vi "DS345 Write.vi"(2 "ON or OFF?":bool[](array[boolean])=[TRUE, TRUE, FALSE], 3 "error in":errorcluster, 4 "Interval Lengths (ms)":dbl[](array[numeric])=[70.0, 30.0, 10.0] format="%.3f", 5 "Arbitrary Waveform Array of Channels (only uses CH 0)":T1(array[cluster])=[[{"AC Frequency (kHz)"=10.0, " Initial AC Ampl. (p-p/2)"=5.0, "Final AC Ampl."=0.0, "Initial DC Value"=-0.1, "Final DC Value"=-0.04, "Constant"=240.0, "Gamma AC"=1.0, "String"="Channel 0 A", "Gamma DC"=0.0}, {"AC Frequency (kHz)"=10.0, " Initial AC Ampl. (p-p/2)"=0.0, "Final AC Ampl."=0.0, "Initial DC Value"=-0.1, "Final DC Value"=-0.04, "Constant"=240.0, "Gamma AC"=1.0, "String"="Channel 0 B", "Gamma DC"=0.0}, {"AC Frequency (kHz)"=10.0, " Initial AC Ampl. (p-p/2)"=0.0, "Final AC Ampl."=0.0, "Initial DC Value"=-0.1, "Final DC Value"=-0.04, "Constant"=240.0, "Gamma AC"=1.0, "String"="Channel 0 C", "Gamma DC"=0.0}], [{"AC Frequency (kHz)"=10.0, " Initial AC Ampl. (p-p/2)"=5.0, "Final AC Ampl."=0.0, "Initial DC Value"=-0.1, "Final DC Value"=-0.04, "Constant"=240.0, "Gamma AC"=1.0, "String"="Channel 1 A", "Gamma DC"=0.0}, {"AC Frequency (kHz)"=10.0, " Initial AC Ampl. (p-p/2)"=0.0, "Final AC Ampl."=0.0, "Initial DC Value"=-0.1, "Final DC Value"=-0.04, "Constant"=199.2, "Gamma AC"=1.0, "String"="Channel 1 B", "Gamma DC"=0.0}, {"AC Frequency (kHz)"=10.0, " Initial AC Ampl. (p-p/2)"=0.0, "Final AC Ampl."=0.0, "Initial DC Value"=-0.1, "Final DC Value"=-0.04, "Constant"=199.2, "Gamma AC"=1.0, "String"="Channel 1 C", "Gamma DC"=0.0}], [{"AC Frequency (kHz)"=10.0, " Initial AC Ampl. (p-p/2)"=0.0, "Final AC Ampl."=0.0, "Initial DC Value"=-0.1, "Final DC Value"=-0.04, "Constant"=199.2, "Gamma AC"=1.0, "String"="Channel 2 A", "Gamma DC"=0.0}, {"AC Frequency (kHz)"=10.0, " Initial AC Ampl. (p-p/2)"=0.0, "Final AC Ampl."=0.0, "Initial DC Value"=-0.1, "Final DC Value"=-0.04, "Constant"=199.2, "Gamma AC"=1.0, "String"="Channel 2 B", "Gamma DC"=0.0}, {"AC Frequency (kHz)"=10.0, " Initial AC Ampl. (p-p/2)"=0.0, "Final AC Ampl."=0.0, "Initial DC Value"=-0.1, "Final DC Value"=-0.04, "Constant"=199.2, "Gamma AC"=1.0, "String"="Channel 2 C", "Gamma DC"=0.0}], [{"AC Frequency (kHz)"=10.0, " Initial AC Ampl. (p-p/2)"=0.0, "Final AC Ampl."=0.0, "Initial DC Value"=-0.1, "Final DC Value"=-0.04, "Constant"=199.2, "Gamma AC"=1.0, "String"="Channel 3 A", "Gamma DC"=0.0}, {"AC Frequency (kHz)"=10.0, " Initial AC Ampl. (p-p/2)"=0.0, "Final AC Ampl."=0.0, "Initial DC Value"=-0.1, "Final DC Value"=-0.04, "Constant"=199.2, "Gamma AC"=1.0, "String"="Channel 3 B", "Gamma DC"=0.0}, {"AC Frequency (kHz)"=10.0, " Initial AC Ampl. (p-p/2)"=0.0, "Final AC Ampl."=0.0, "Initial DC Value"=-0.1, "Final DC Value"=-0.04, "Constant"=199.2, "Gamma AC"=1.0, "String"="Channel 3 C", "Gamma DC"=0.0}], [{"AC Frequency (kHz)"=10.0, " Initial AC Ampl. (p-p/2)"=0.0, "Final AC Ampl."=0.0, "Initial DC Value"=-0.1, "Final DC Value"=-0.04, "Constant"=199.2, "Gamma AC"=1.0, "String"="Channel 4 A", "Gamma DC"=0.0}, {"AC Frequency (kHz)"=10.0, " Initial AC Ampl. (p-p/2)"=0.0, "Final AC Ampl."=0.0, "Initial DC Value"=-0.1, "Final DC Value"=-0.04, "Constant"=199.2, "Gamma AC"=1.0, "String"="Channel 4 B", "Gamma DC"=0.0}, {"AC Frequency (kHz)"=10.0, " Initial AC Ampl. (p-p/2)"=0.0, "Final AC Ampl."=0.0, "Initial DC Value"=-0.1, "Final DC Value"=-0.04, "Constant"=199.2, "Gamma AC"=1.0, "String"="Channel 4 C", "Gamma DC"=0.0}], [{"AC Frequency (kHz)"=10.0, " Initial AC Ampl. (p-p/2)"=0.0, "Final AC Ampl."=0.0, "Initial DC Value"=-0.1, "Final DC Value"=-0.04, "Constant"=199.2, "Gamma AC"=1.0, "String"="Channel 5 A", "Gamma DC"=0.0}, {"AC Frequency (kHz)"=10.0, " Initial AC Ampl. (p-p/2)"=0.0, "Final AC Ampl."=0.0, "Initial DC Value"=-0.1, "Final DC Value"=-0.04, "Constant"=199.2, "Gamma AC"=1.0, "String"="Channel 5 B", "Gamma DC"=0.0}, {"AC Frequency (kHz)"=10.0, " Initial AC Ampl. (p-p/2)"=0.0, "Final AC Ampl."=0.0, "Initial DC Value"=-0.1, "Final DC Value"=-0.04, "Constant"=199.2, "Gamma AC"=1.0, "String"="Channel 5 C", "Gamma DC"=0.0}], [{"AC Frequency (kHz)"=10.0, " Initial AC Ampl. (p-p/2)"=0.0, "Final AC Ampl."=0.0, "Initial DC Value"=-0.1, "Final DC Value"=-0.04, "Constant"=199.2, "Gamma AC"=1.0, "String"="Channel 6 A", "Gamma DC"=0.0}, {"AC Frequency (kHz)"=10.0, " Initial AC Ampl. (p-p/2)"=0.0, "Final AC Ampl."=0.0, "Initial DC Value"=-0.1, "Final DC Value"=-0.04, "Constant"=199.2, "Gamma AC"=1.0, "String"="Channel 6 B", "Gamma DC"=0.0}, {"AC Frequency (kHz)"=10.0, " Initial AC Ampl. (p-p/2)"=0.0, "Final AC Ampl."=0.0, "Initial DC Value"=-0.1, "Final DC Value"=-0.04, "Constant"=199.2, "Gamma AC"=1.0, "String"="Channel 6 C", "Gamma DC"=0.0}], [{"AC Frequency (kHz)"=10.0, " Initial AC Ampl. (p-p/2)"=0.0, "Final AC Ampl."=0.0, "Initial DC Value"=-0.1, "Final DC Value"=-0.04, "Constant"=199.2, "Gamma AC"=1.0, "String"="Channel 7 A", "Gamma DC"=0.0}, {"AC Frequency (kHz)"=10.0, " Initial AC Ampl. (p-p/2)"=0.0, "Final AC Ampl."=0.0, "Initial DC Value"=-0.1, "Final DC Value"=-0.04, "Constant"=199.2, "Gamma AC"=1.0, "String"="Channel 7 B", "Gamma DC"=0.0}, {"AC Frequency (kHz)"=10.0, " Initial AC Ampl. (p-p/2)"=0.0, "Final AC Ampl."=0.0, "Initial DC Value"=-0.1, "Final DC Value"=-0.04, "Constant"=199.2, "Gamma AC"=1.0, "String"="Channel 7 C", "Gamma DC"=0.0}]] {"Gamma DC" format="%.2f"; "Gamma AC" format="%.2f"; "Constant" min=0.0 max=240.0 format="%.2f"; "Final DC Value" format="%.3f"; "Initial DC Value" format="%.3f"; "Final AC Ampl." format="%.3f"; "Initial AC Ampl. (p-p/2)" format="%.3f"; "AC Frequency (kHz)" format="%.2f"}) -> (0 "error out":errorcluster, 1 "Waveform (dither)":cluster{dbl[], dbl[]}(graph))   [LabVIEW 2013]
panel:
  in  "Case Constant\n(See Context Help)":bool=TRUE
  out "Actual used channels":bool[](array[boolean])
  out "Array":dbl[](array[numeric]) format="%^.5e"
  out "log2(x)":dbl format="%.2f"
  out "ceil(x): smallest int >= x":dbl format="%.2f"
  out "Est. Sampling Rate":dbl format="%.2f"
  out "Total Waveform Time":dbl format="%.2f"
  out "Number of points":dbl=16000.0 format="%.2f"
  out "Sampling Rate":dbl=160000.0 format="%.2f"
  in  "trigger rate":ext=100.0 format="%.3f"
  in  "Memory Address (0 to 9)\n(stores waveform)":string="0"
  in  "trigger source (single:0)":i32(ring)=2 items=["single", "internal rate", "+ slope external", "- slope external", "line"]
  in  "ARB.wave source":u16(ring)=1 items=[".WAV file", "array in point mode", "array in vector mode"]
  in  "single trigger":bool
  in  "FREQ. units (Hz:0)":i32(ring) items=["Hz", "KHz.", "MHz."]
  in  "phase":ext format="%.3f"
  in  "DC offset":ext format="%.3f"
  in  "amplitude (0 Vrms:0)":cluster{ext, i32}={1.0, 1} {"?" items=["Vrms", "Vpp", "dBm"]; "?" format="%.3f"}
  in  "frequency":ext=555.0 format="%.6f"
  in  "output function (sine:0)":u16(ring)=5 items=["sine", "square", "triangle", "ramp", "noise", "arbitrary"]
  in  "Command to Send":string="*RST;"
  in  "GPIB Address":string="19"
  # "DS 345 Settings"
  # "Note that Interval C is disabled for DS345"
  # "Sampling Rate of DS345\nDefaults to Closest Value \n(up or down) of \n40MHz/n where n is a\npositive integer."
  # "Interval A"
  # "Interval B"
  # "Interval C"
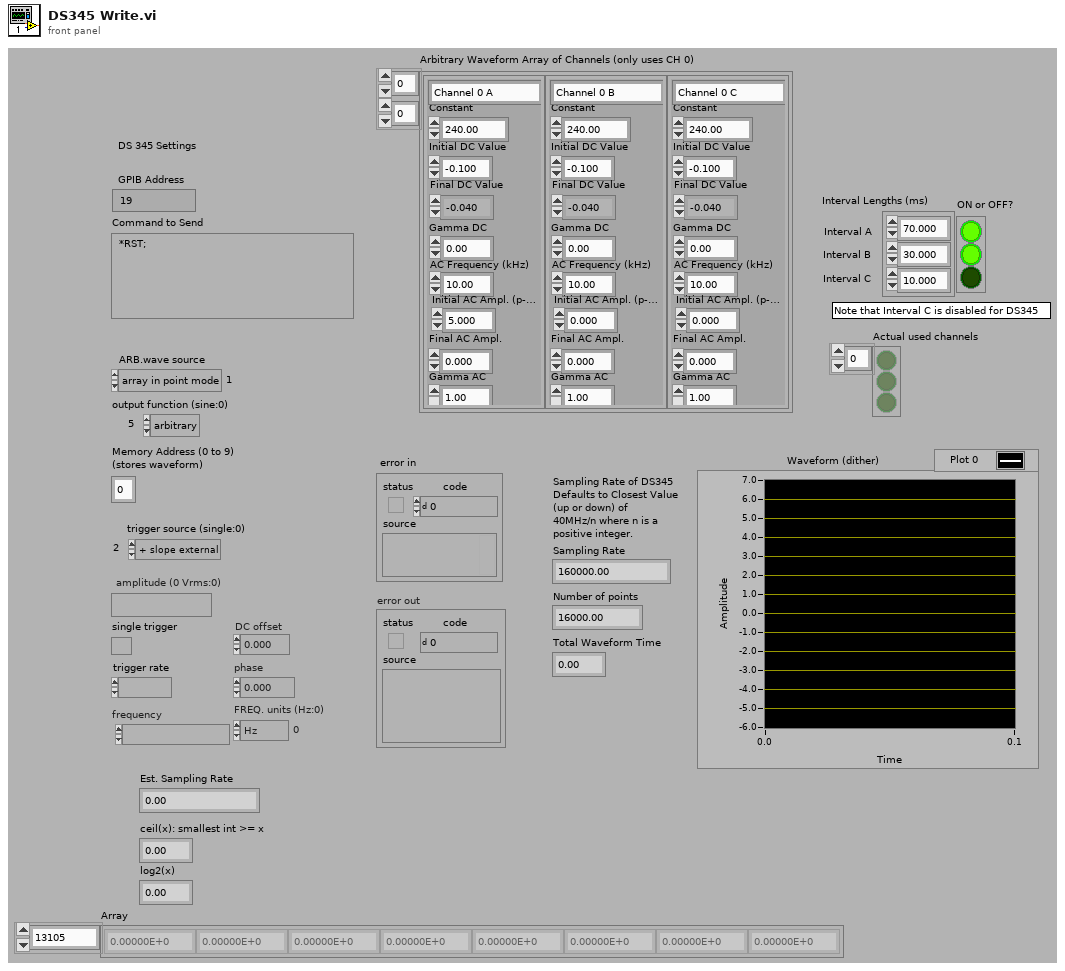
[diagram p1: front panel]
types:
  T1 = cluster{"AC Frequency (kHz)":dbl, " Initial AC Ampl. (p-p/2)":dbl, "Final AC Ampl.":dbl, "Initial DC Value":dbl, "Final DC Value":dbl, "Constant":dbl, "Gamma AC":dbl, "String":string, "Gamma DC":dbl}[][]
  T2 = cluster{"AC Frequency (kHz)":dbl, " Initial AC Ampl. (p-p/2)":dbl, "Final AC Ampl.":dbl, "Initial DC Value":dbl, "Final DC Value":dbl, "Constant":dbl, "Gamma AC":dbl, "String":string, "Gamma DC":dbl}[]
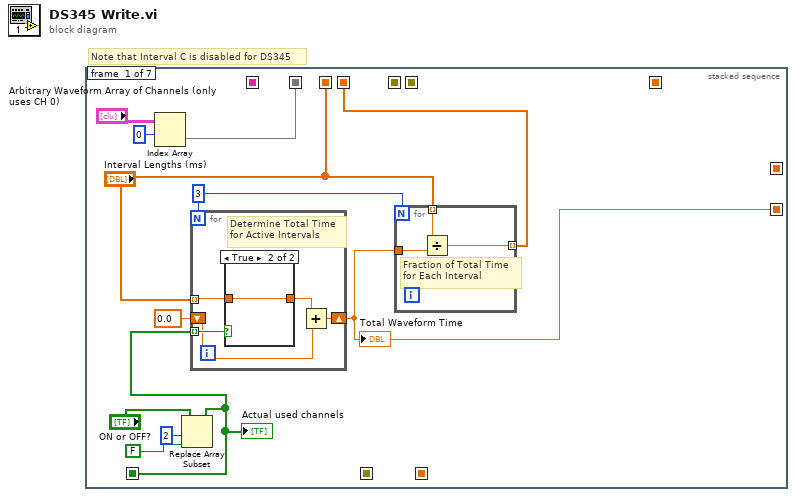
[diagram p0: block diagram]
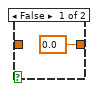
[diagram p2: hidden frame]
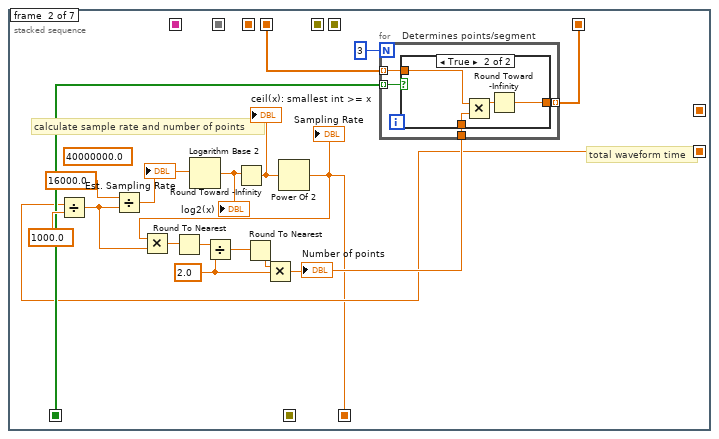
[diagram p3: hidden frame]
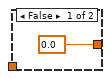
[diagram p4: hidden frame]
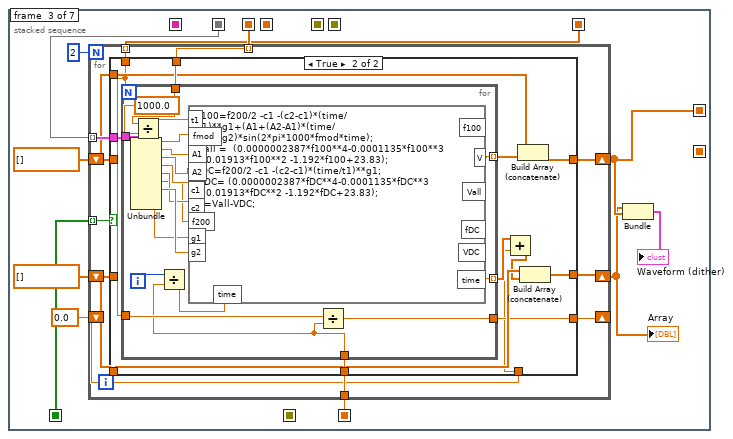
[diagram p5: hidden frame]
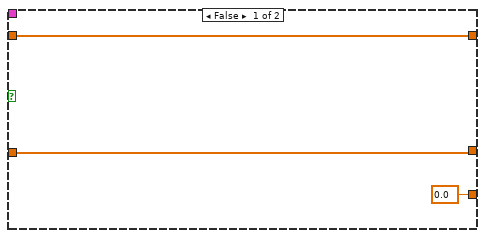
[diagram p6: hidden frame]
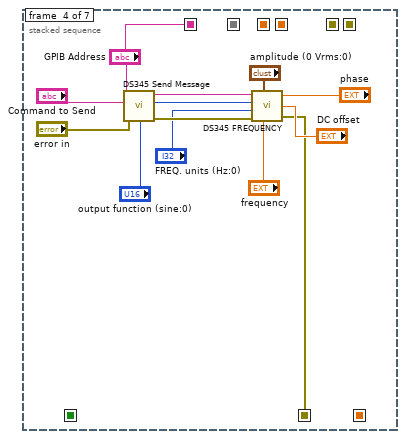
[diagram p7: hidden frame]
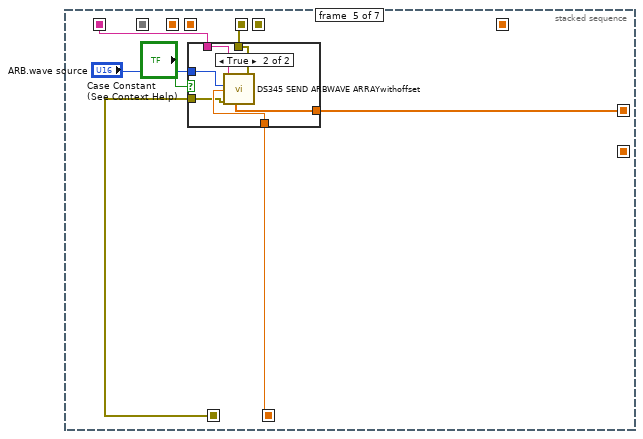
[diagram p8: hidden frame]
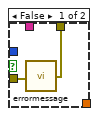
[diagram p9: hidden frame]
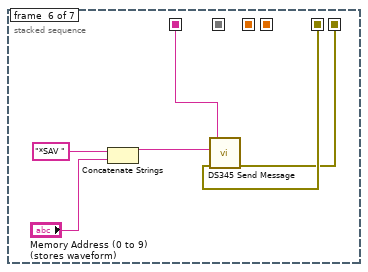
[diagram p10: hidden frame]
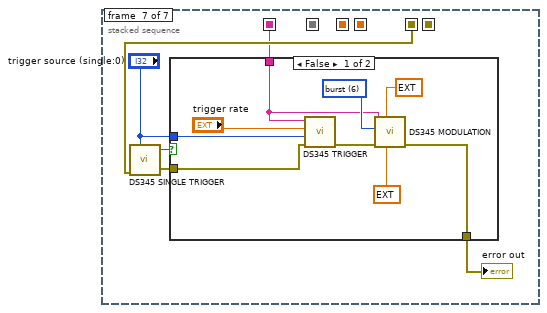
[diagram p11: hidden frame]
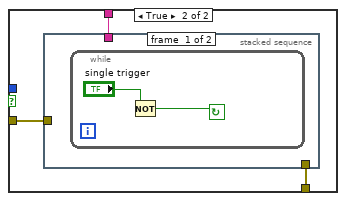
[diagram p12: hidden frame]
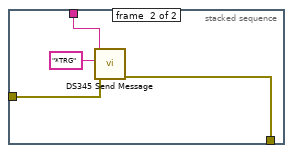
[diagram p13: hidden frame]
diagram:
  # "Note that Interval C is disabled for DS345"
  n1 = stacked-sequence {
    seq-local: [_ _ _ _ w125 _ _] -> [_ _ _ _ _ w137 w145]
    seq-local: [_ _ _ _ _ w136 _] -> [_ _ _ _ _ _ _]
    seq-local: [_ w23 _ _ _ _ _] -> [_ _ w61 _ w120 _ _]
    seq-local: [_ _ w52 _ _ _ _] -> [_ _ _ _ w121 _ _]
    seq-local: [_ _ _ "GPIB Address" _ _ _] -> [_ _ _ _ w123 w135 w142]
    seq-local: [_ _ _ w108 _ _ _] -> [_ _ _ _ w122 _ _]
    seq-local: [w11 _ _ _ _ _ _] -> [_ _ w60 _ _ _ _]
    seq-local: [w5 _ _ _ _ _ _] -> [_ w28 _ _ _ _ _]
    seq-local: ["Interval Lengths (ms)" _ _ _ _ _ _] -> [_ _ w59 _ _ _ _]
    seq-local: [w6 _ _ _ _ _ _] -> [_ w30 _ _ _ _ _]
    seq-local: [_ w31 _ _ _ _ _] -> [_ _ w58 _ _ _ _]
    seq-local: [w1 _ _ _ _ _ _] -> [_ w32 w56 _ _ _ _]
    frame #0 {
      w9 = 3
      n2 = Index Array(array="Arbitrary Waveform Array of Channels (only uses CH 0)", index (row)=0) -> (element=w11:T2)  [unwired: 1 in]
      n3 = Replace Array Subset(array="ON or OFF?", new element=FALSE ("new element/subarray"), index=2) -> (w1:bool[])
      "Actual used channels" <- w1
      n4 = for {
        N: w9 -> [_]
        tunnel: w1 -> [w20] mode=indexing
        tunnel: "Interval Lengths (ms)" -> [w19] mode=indexing
        shift-right: [w17] -> w5
        shift-left: 0.0 -> [w16]
        # "Determine Total Time\nfor Active Intervals"
        n5 = case shown="True" w20 {
          tunnel: w19 -> [_ w22]
          tunnel: [0.0 ("Interval A (ms)") w22] -> w18
          frame False {
          }
          frame True {
          }
        }
        n6 = Add(x=w18, y=w16) -> (x+y=w17:dbl)
      }
      "Total Waveform Time" <- w5
      n7 = for {
        N: w9 -> [_]
        tunnel: "Interval Lengths (ms)" -> [w15] mode=indexing
        tunnel: w5 -> [w14]
        tunnel: [w13] -> w6 mode=indexing
        # "Fraction of Total Time\nfor Each Interval"
        n8 = Divide(x=w15, y=w14) -> (x/y=w13:dbl)
      }
    }
    frame #1 {
      w34 = 2.0 ("y")
      (unwired) 40000000.0 ("x")
      # "total waveform time"
      # "calculate sample rate and number of points"
      n9 = Divide(x=w28, y=1000.0 ("10000")) -> (x/y=w27:dbl)
      n10 = Divide(x=16000.0, y=w27) -> (x/y=w26:dbl)
      "Est. Sampling Rate" <- w26
      n11 = Logarithm Base 2(1:w26) -> (0:w25:dbl)
      "log2(x)" <- w25
      n12 = Round Toward -Infinity(1:w25) -> (0:w24:dbl)
      "ceil(x): smallest int >= x" <- w24
      n13 = Power Of 2(x=w24) -> (2^x=w23:dbl)
      "Sampling Rate" <- w23
      n14 = Multiply(x=w23, y=w27) -> (x*y=w38:dbl)
      n15 = Round To Nearest(number=w38) -> (nearest integer value=w37:dbl)
      n16 = Divide(x=w37, y=w34) -> (x/y=w36:dbl)
      n17 = Round To Nearest(number=w36) -> (nearest integer value=w35:dbl)
      n18 = Multiply(x=w35, y=w34) -> (x*y=w33:dbl)
      "Number of points" <- w33
      n19 = for "Determines points/segment" {
        N: 3 -> [_]
        tunnel: w32 -> [w44] mode=indexing
        tunnel: [w43] -> w31 mode=indexing
        tunnel: w33 -> [w42]
        tunnel: w30 -> [w41] mode=indexing
        n20 = case shown="True" w44 {
          tunnel: [0.0 w49] -> w43
          tunnel: w42 -> [_ w47]
          tunnel: w41 -> [_ w46]
          frame False {
          }
          frame True {
            n21 = Multiply(x=w46, y=w47) -> (x*y=w48:dbl)
            n22 = Round Toward -Infinity(1:w48) -> (0:w49:dbl)
          }
        }
      }
    }
    frame #2 {
      n23 = for {
        N: 2 -> [_]
        tunnel: w61 -> [w72]
        tunnel: w60 -> [w71] mode=indexing
        tunnel: w59 -> [w70] mode=indexing
        tunnel: w58 -> [w69] mode=indexing
        tunnel: w56 -> [w68] mode=indexing
        shift-right: [w67] -> w52
        shift-left: dbl[] [] -> [w66]
        shift-right: [w65] -> w51
        shift-left: dbl[] [] -> [w64]
        shift-right: [w63] -> _
        shift-left: 0.0 -> [w62]
        n24 = case shown="True" w68 {
          tunnel: w72 -> [_ w88]
          tunnel: w71 -> [_ w87]
          tunnel: w70 -> [_ w86]
          tunnel: w69 -> [_ w80]
          tunnel: [w75 w84] -> w67
          tunnel: w66 -> [_ w83]
          tunnel: w66 -> [w75 _]
          tunnel: [w74 w82] -> w65
          tunnel: w64 -> [_ w81]
          tunnel: w64 -> [w74 _]
          tunnel: [0.0 w79] -> w63
          tunnel: w62 -> [_ w77]
          frame False {
          }
          frame True {
            n25 = for {
              N: w80 -> [_]
              tunnel: w88 -> [w90]
              tunnel: w87 -> [w106]
              tunnel: w86 -> [w102]
              tunnel: [w97] -> w85 mode=indexing
              tunnel: [w96] -> w78 mode=indexing
              tunnel: w80 -> [w91]
              tunnel: [w89] -> w79
              i -> [w107]
              n26 = Unbundle(w106) -> ("AC Frequency (kHz)"=w98:dbl, "Initial AC Ampl. (p-p/2)"=w99:dbl, "Final AC Ampl."=w100:dbl, "Initial DC Value"=w95:dbl, "Final DC Value"=w94:dbl, "Constant"=w93:dbl, "Gamma AC"=w101:dbl, "Gamma DC"=w92:dbl)  [unwired: 1 out]
              n27 = Divide(x=w102, y=1000.0) -> (x/y=w103:dbl)
              n28 = Divide(x=w107, y=w90) -> (x/y=w105:dbl)
              n29 = formula code="f100=f200/2 -c1 -(c2-c1)*(time/t1)**g1+(A1+(A2-A1)*(time/t1)**g2)*sin(2*pi*1000*fmod*time);\nVall =  (0.0000002387*f100**4-0.0001135*f100**3 +0.01913*f100**2 -1.192*f100+23.83);\nfDC=f200/2 -c1 -(c2-c1)*(time/t1)**g1;\nVDC= (0.0000002387*fDC**4-0.0001135*fDC**3 +0.01913*fDC**2 -1.192*fDC+23.83);\nV=Vall-VDC;"("c1"=w95, "time"=w105, "t1"=w103, "c2"=w94, "f200"=w93, "fmod"=w98, "A1"=w99, "A2"=w100, "g1"=w92, "g2"=w101) -> ("time"=w96:dbl, "V"=w97:dbl)  [unwired: 4 out]
              n30 = Divide(x=w91, y=w90) -> (x/y=w89:dbl)
            }
            n31 = Add(x=w78, y=w77) -> (x+y=w76:dbl[])
            n32 = Build Array (concatenate)(w83, w85) -> (w84:dbl[])
            n33 = Build Array (concatenate)(w81, w76) -> (w82:dbl[])
          }
        }
      }
      "Array" <- w51
      n34 = Bundle(w51, w52) -> (→"Waveform (dither)":cluster{dbl[], dbl[]})  [unwired: 1 in]
    }
    frame #3 {
      n35 = call "DS345 Send Message.vi"("address string"="GPIB Address", "write buffer"="Command to Send", "error in"="error in") -> ("address out"=w110:string, "error out"=w114:errorcluster)  [unwired: 3 in, 2 out]
      n36 = call "DS345 FREQUENCY.vi"("GPIB address"=w110, "amplitude (0 Vrms:0)"="amplitude (0 Vrms:0)", "output function (sine:0)"="output function (sine:0)", "FREQ. units (Hz:0)"="FREQ. units (Hz:0)", "frequency"="frequency", "error in"=w114, "phase"="phase", "DC offset"="DC offset") -> ("error out"=w108:errorcluster)
    }
    frame #4 {
      n37 = case shown="True" "Case Constant\n(See Context Help)" {
        tunnel: "ARB.wave source" -> [_ w134]
        tunnel: w123 -> [_ w133]
        tunnel: [w128 w132] -> w125
        tunnel: w120 -> [_ w131]
        tunnel: w122 -> [w127 w130]
        tunnel: w121 -> [_ w129]
        frame False {
          n38 = call "errormessage.vi"("error in"=w127) -> ("error out"=w128:errorcluster)
        }
        frame True {
          n39 = call "DS345 SEND ARBWAVE ARRAYwithoffset.VI"("y vertices / amplitude points"=w129, "error in"=w130, "sampling FREQ."=w131, "ARB.wave source"=w134, "GPIB address"=w133) -> ("error out"=w132:errorcluster)  [unwired: 1 in]
        }
      }
    }
    frame #5 {
      n40 = Concatenate Strings("*SAV " ("string"), "Memory Address (0 to 9)\n(stores waveform)") -> (w138:string)
      n41 = call "DS345 Send Message.vi"("address string"=w135, "write buffer"=w138, "error in"=w137) -> ("error out"=w136:errorcluster)  [unwired: 3 in, 3 out]
    }
    frame #6 {
      n42 = call "DS345 SINGLE TRIGGER.VI"("error in"=w145, "trigger source (single:0)"="trigger source (single:0)") -> ("error out"=w141:errorcluster, "single trigger"=w146:bool)  [unwired: 2 in]
      n43 = case shown="False" w146 {
        tunnel: w141 -> [w147 w158]
        tunnel: "trigger source (single:0)" -> [w155 _]
        tunnel: [w149 w157] -> w143
        tunnel: w142 -> [w148 w156]
        frame False {
          w151 = 6 items=["off", "linear sweep", "log sweep", "amplitude", "frequency", "phase ", "burst"] ("modulation(off:0)")
          n44 = call "DS345 TRIGGER.VI"("GPIB  address"=w148, "trigger rate"="trigger rate", "trigger source (single:0)"=w155, "error in"=w147) -> ("error out"=w153:errorcluster)  [unwired: 1 in]
          n45 = call "DS345 MODULATION.VI"("span/depth/\nburst count"=ext 1.0 ("span/depth/\nburst count"), "modulation rate"=ext 1.0, "error in"=w153, "modulation(off:0)"=w151, "GPIB  address"=w148) -> ("error out"=w149:errorcluster)  [unwired: 6 in]
        }
        frame True {
          n46 = stacked-sequence {
            tunnel: w158 -> [_ w163]
            tunnel: [_ w162] -> w157
            tunnel: w156 -> [_ w161]
            frame #0 {
              n47 = while {
                stop <- w160 continue-if-true
                n48 = Not(x="single trigger") -> (.not. x?=w160:bool)
              }
            }
            frame #1 {
              n49 = call "DS345 Send Message.vi"("address string"=w161, "write buffer"="*TRG", "error in"=w163) -> ("error out"=w162:errorcluster)  [unwired: 3 in, 3 out]
            }
          }
        }
      }
      "error out" <- w143
    }
  }
